vi "power_meas.vi"() -> ()   [LabVIEW 2019]
uses:
  <vilib>/Utility/error.llb/DialogType.ctl
  <vilib>/DAQmx/write.llb/DAQmx Write (Digital Bool 1Line 1Point).vi
  <vilib>/DAQmx/write.llb/DAQmx Write (Counter Frequency 1Chan 1Samp).vi
  <vilib>/DAQmx/miscellaneous.llb/DAQmx Fill In Error Info.vi
  <vilib>/DAQmx/create/channels.llb/DAQmx Create Channel (CO-Pulse Generation-Frequency).vi
  <vilib>/DAQmx/configure/timing.llb/DAQmx Timing (Implicit).vi
  <vilib>/addons/control/pid/pid.llb/PID (DBL).vi
  <vilib>/Utility/file.llb/Write Delimited Spreadsheet (string).vi
  <instrlib>/Agilent 34970/Agilent 34970.lvlib
  <resource>/objmgr/daqmx.rc
  <vilib>/addons/control/pid/NI_PID_pid.lvlib
  <instrlib>/Yokogawa WT200 Series/Yokogawa WT200 Series.lvlib
panel:
  in  "Idenfier_Ens. Term.":string="medsETMA"
  out "TP 15":dbl
  out "TP 13":dbl
  out "TP 12":dbl
  out "TP 11":dbl
  out "TP 10":dbl
  out "TP 8":dbl
  out "TP 7":dbl
  out "TP 6":dbl
  out "TP 5":dbl
  out "TP 3":dbl
  out "TP 2":dbl
  out "TP 1":dbl
  in  "Idenfier_Freio":string="medsFreio"
  in  "Identifier_Watt":string="medsWatt"
  out "PL(E)":dbl
  out "PC(E)":dbl
  out "PC(T)":dbl
  out "PL(T)":dbl
  out "t":dbl
  out "Tensão de saída":dbl format="%.4f"
  out "Corrente de saída":dbl format="%.4f"
  out "watt num cluster":T1
  in  "Liga Fonte":bool
  out "Resposta":string
  out "Tradução":string
  in  "Parar motor":bool
  in  "Envia mensagem":bool
  in  "Enviar velocidade":bool
  in  "Seta carga":bool
  in  "Limite de tensão":dbl=17.0 min=0.0 max=17.0 step=0.5 format="%.4f"
  in  "Limite de corrente":dbl=0.075 min=0.0 max=0.4 step=0.01 format="%.4f"
  in  "Mensagem":T2(ring)=enum."Read power"
  in  "Velocidade (RPM)":u16=1000 min=1000 max=10000 step=100
  in  "Parâmetros serial":T3={"Serial VCC"="COM7", "timeout"=2, "baud rate"=600, "flow control"=0, "data bits"=8, "parity"=enum."None", "stop bits"=10, "termination char"=FALSE} {"stop bits" items=["1.0"=10, "1.5"=15, "2.0"=20]; "flow control" items=["None", "XON/XOFF", "RTS/CTS", "XON/XOFF & RTS/CTS", "DTR/DSR", "XON/XOFF & DTR/DSR"]}
  in  "Medição contínua? WT230":bool=TRUE
  in  "Realiza medição WT230":bool=TRUE
  out "Chart potencia numeric":T4(graph)
  out "Chart corrente numeric":cluster{"I(A)":dbl, "I(B)":dbl, "I(E)":dbl}(graph)
  out "Chart tensão numeric":cluster{"V(A)":dbl, "V(B)":dbl, "V(E)":dbl}(graph)
  in  "Tempo de integração (s)":u32=5 min=1 max=60 step=1
  in  "SP:":dbl(slide)=25.0 min=0.0 max=0.0 scale=25.0..50.0
  out "MV":dbl(graph)
  in  "Ts":dbl=1.0
  out "PV":dbl
  out "Process variable and Setpoint":cluster{"initial PV":dbl, "SP:":dbl}(graph)
  in  "PID gains":T5={"proportional gain (Kc)"=39.6, "integral time (Ti, min)"=14.617, "derivative time (Td, min)"=0.0} {"derivative time (Td, min)" format="%.3f"; "integral time (Ti, min)" format="%.3f"; "proportional gain (Kc)" format="%.6f"}
  in  "Frequency":dbl=1.0 format="%.6f"
  out "Duty Cycle":sgl=0.1 min=0.1 max=99.9 format="%#_6f"
  in  "Forno_on":bool=TRUE
  out "Iteration":i32
  out "Chart PV, SP":cluster{dbl, dbl}(graph)
  in  "STOP":bool
  out "Temperature CH4 [degC]":dbl
  out "Temperature CH9 [degC]":dbl
  out "Time":dbl=300.0 format="%<%H:%M:%S>t"
  in  "Idenfier_Forno":string="medsForno"
  # "Temperaturas dos Termopares"
  # "Controle de Temperatura do Forno"
  # "Freio"
  # "Wattímetro WT230 Yokogawa"
  # "Geral"
  # "Respostas do Sistema em Malha Fechada"
  # "Controles"
  # "Controles"
  # "Medidas"
  # "Respostas temporais"
  # "Medidas"
  # "Controles"
  # "Inversor de Frequência"
  # "Comandos"
  # "Medidas"
  # "Parâmetros Serial"
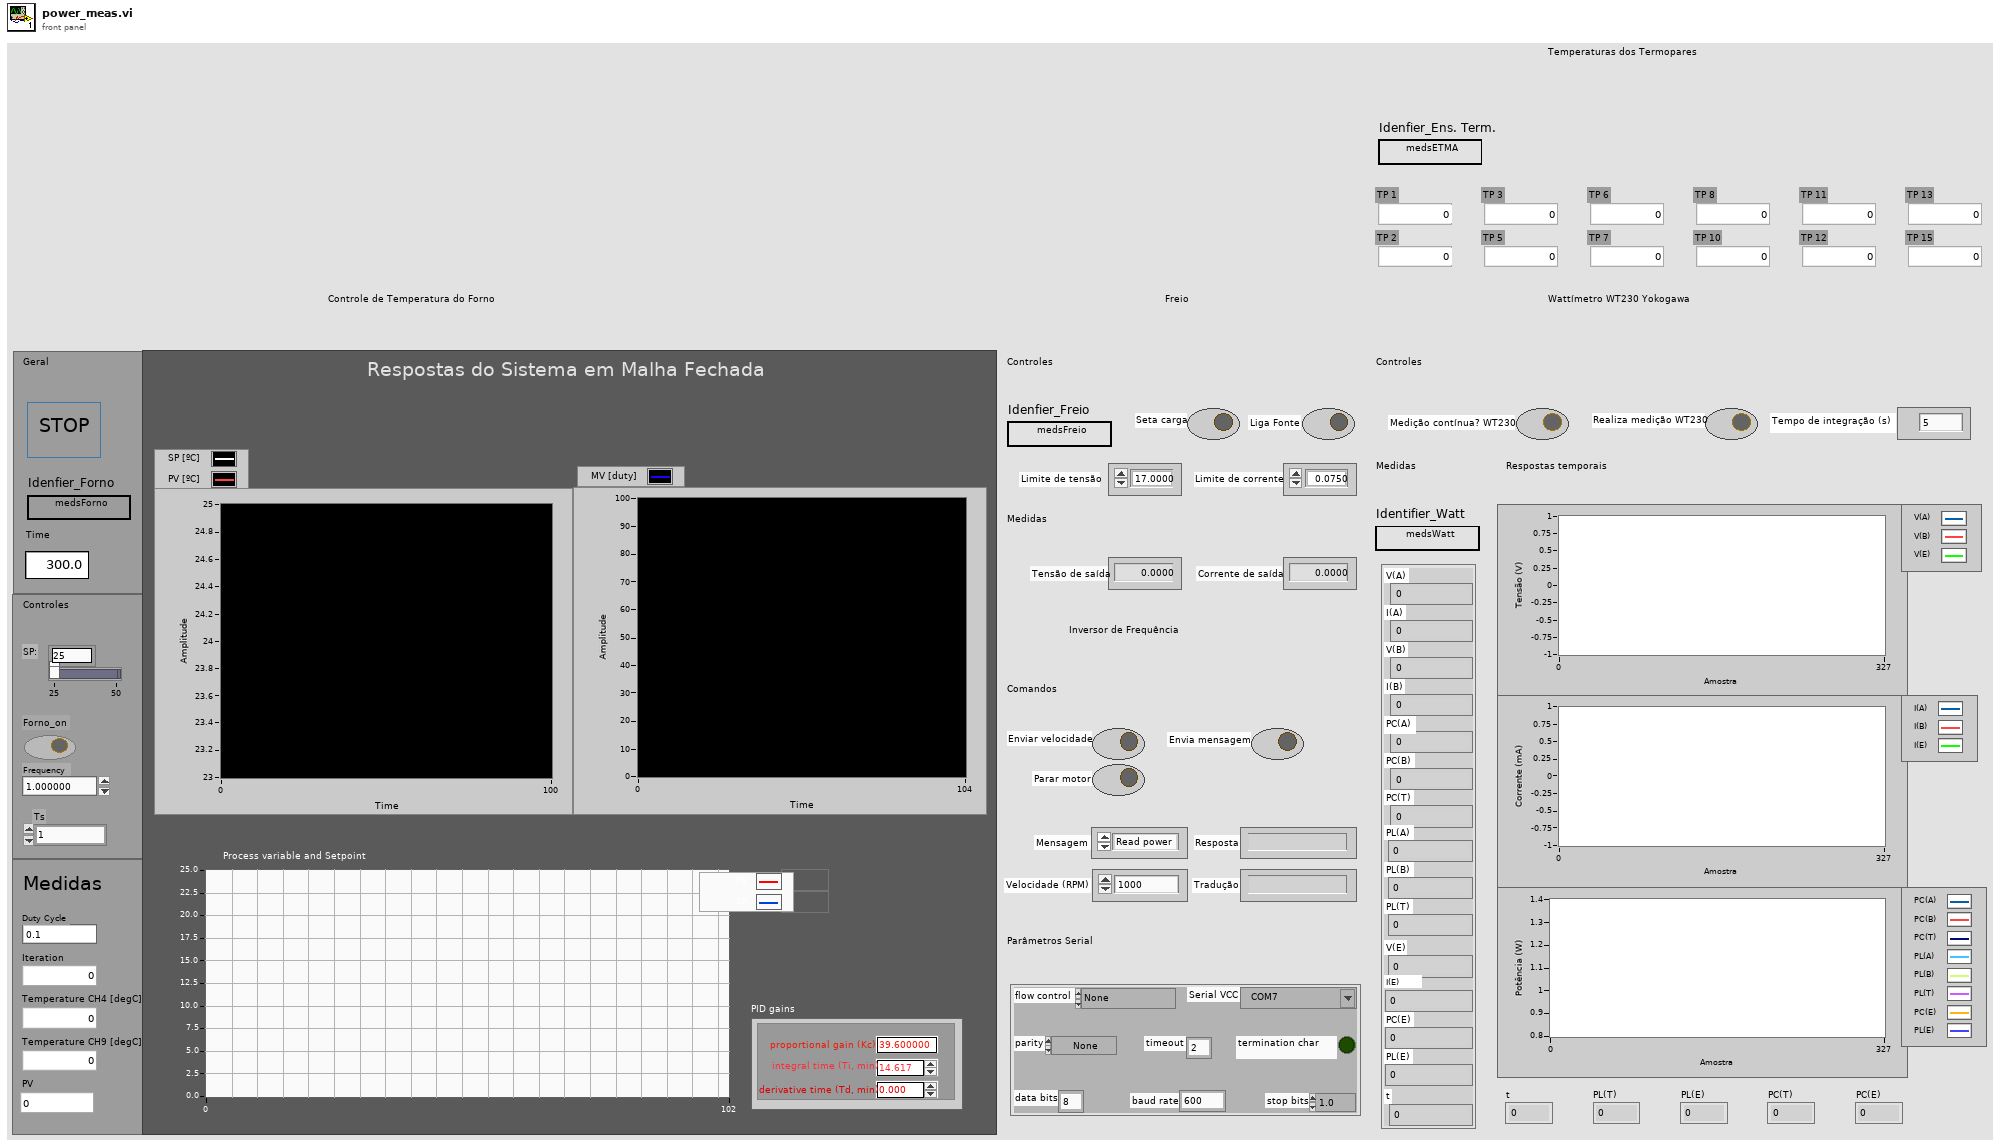
[diagram p1: front panel]
types:
  T1 = cluster{"V(A)":dbl, "I(A)":dbl, "V(B)":dbl, "I(B)":dbl, "PC(A)":dbl, "PC(B)":dbl, "PC(T)":dbl, "PL(T)":dbl, "PL(B)":dbl, "PL(A)":dbl, "V(E)":dbl, "PL(E)":dbl, "PC(E)":dbl, "I(E)":dbl, "t":dbl}
  T2 = enum16{"Read set speed", "Read operation status", "Read power", "Read starting trials", "Read bus voltage", "Read temperature", "Read power limitation", "Read PWM mode", "Read PWM frequency", "Read real speed"}
  T3 = cluster{"Serial VCC":refnum<visa-resource-name>, "timeout":u32, "baud rate":u32, "flow control":u16, "data bits":u16, "parity":enum16{"None", "Odd", "Even", "Mark", "Space"}, "stop bits":u16, "termination char":bool}
  T4 = cluster{"PC(A)":dbl, "PC(B)":dbl, "PC(T)":dbl, "PL(A)":dbl, "PL(B)":dbl, "PL(T)":dbl, "PC(E)":dbl, "PL(E)":dbl}
  T5 = cluster{"proportional gain (Kc)":dbl, "integral time (Ti, min)":dbl, "derivative time (Td, min)":dbl}
  T6 = enum16{"Start Comm.", "End Comm.", "Wait", "Send Static Message", "Set Speed"}
  T7 = enum16{"Thermocouple", "Thermistor", "RTD", "4-Wire RTD", "Default (Last)"}
  T8 = enum8{"Enabled", "Disabled", "Disabled and Grayed Out"}
  T9 = typedef "DialogType.ctl" = u16
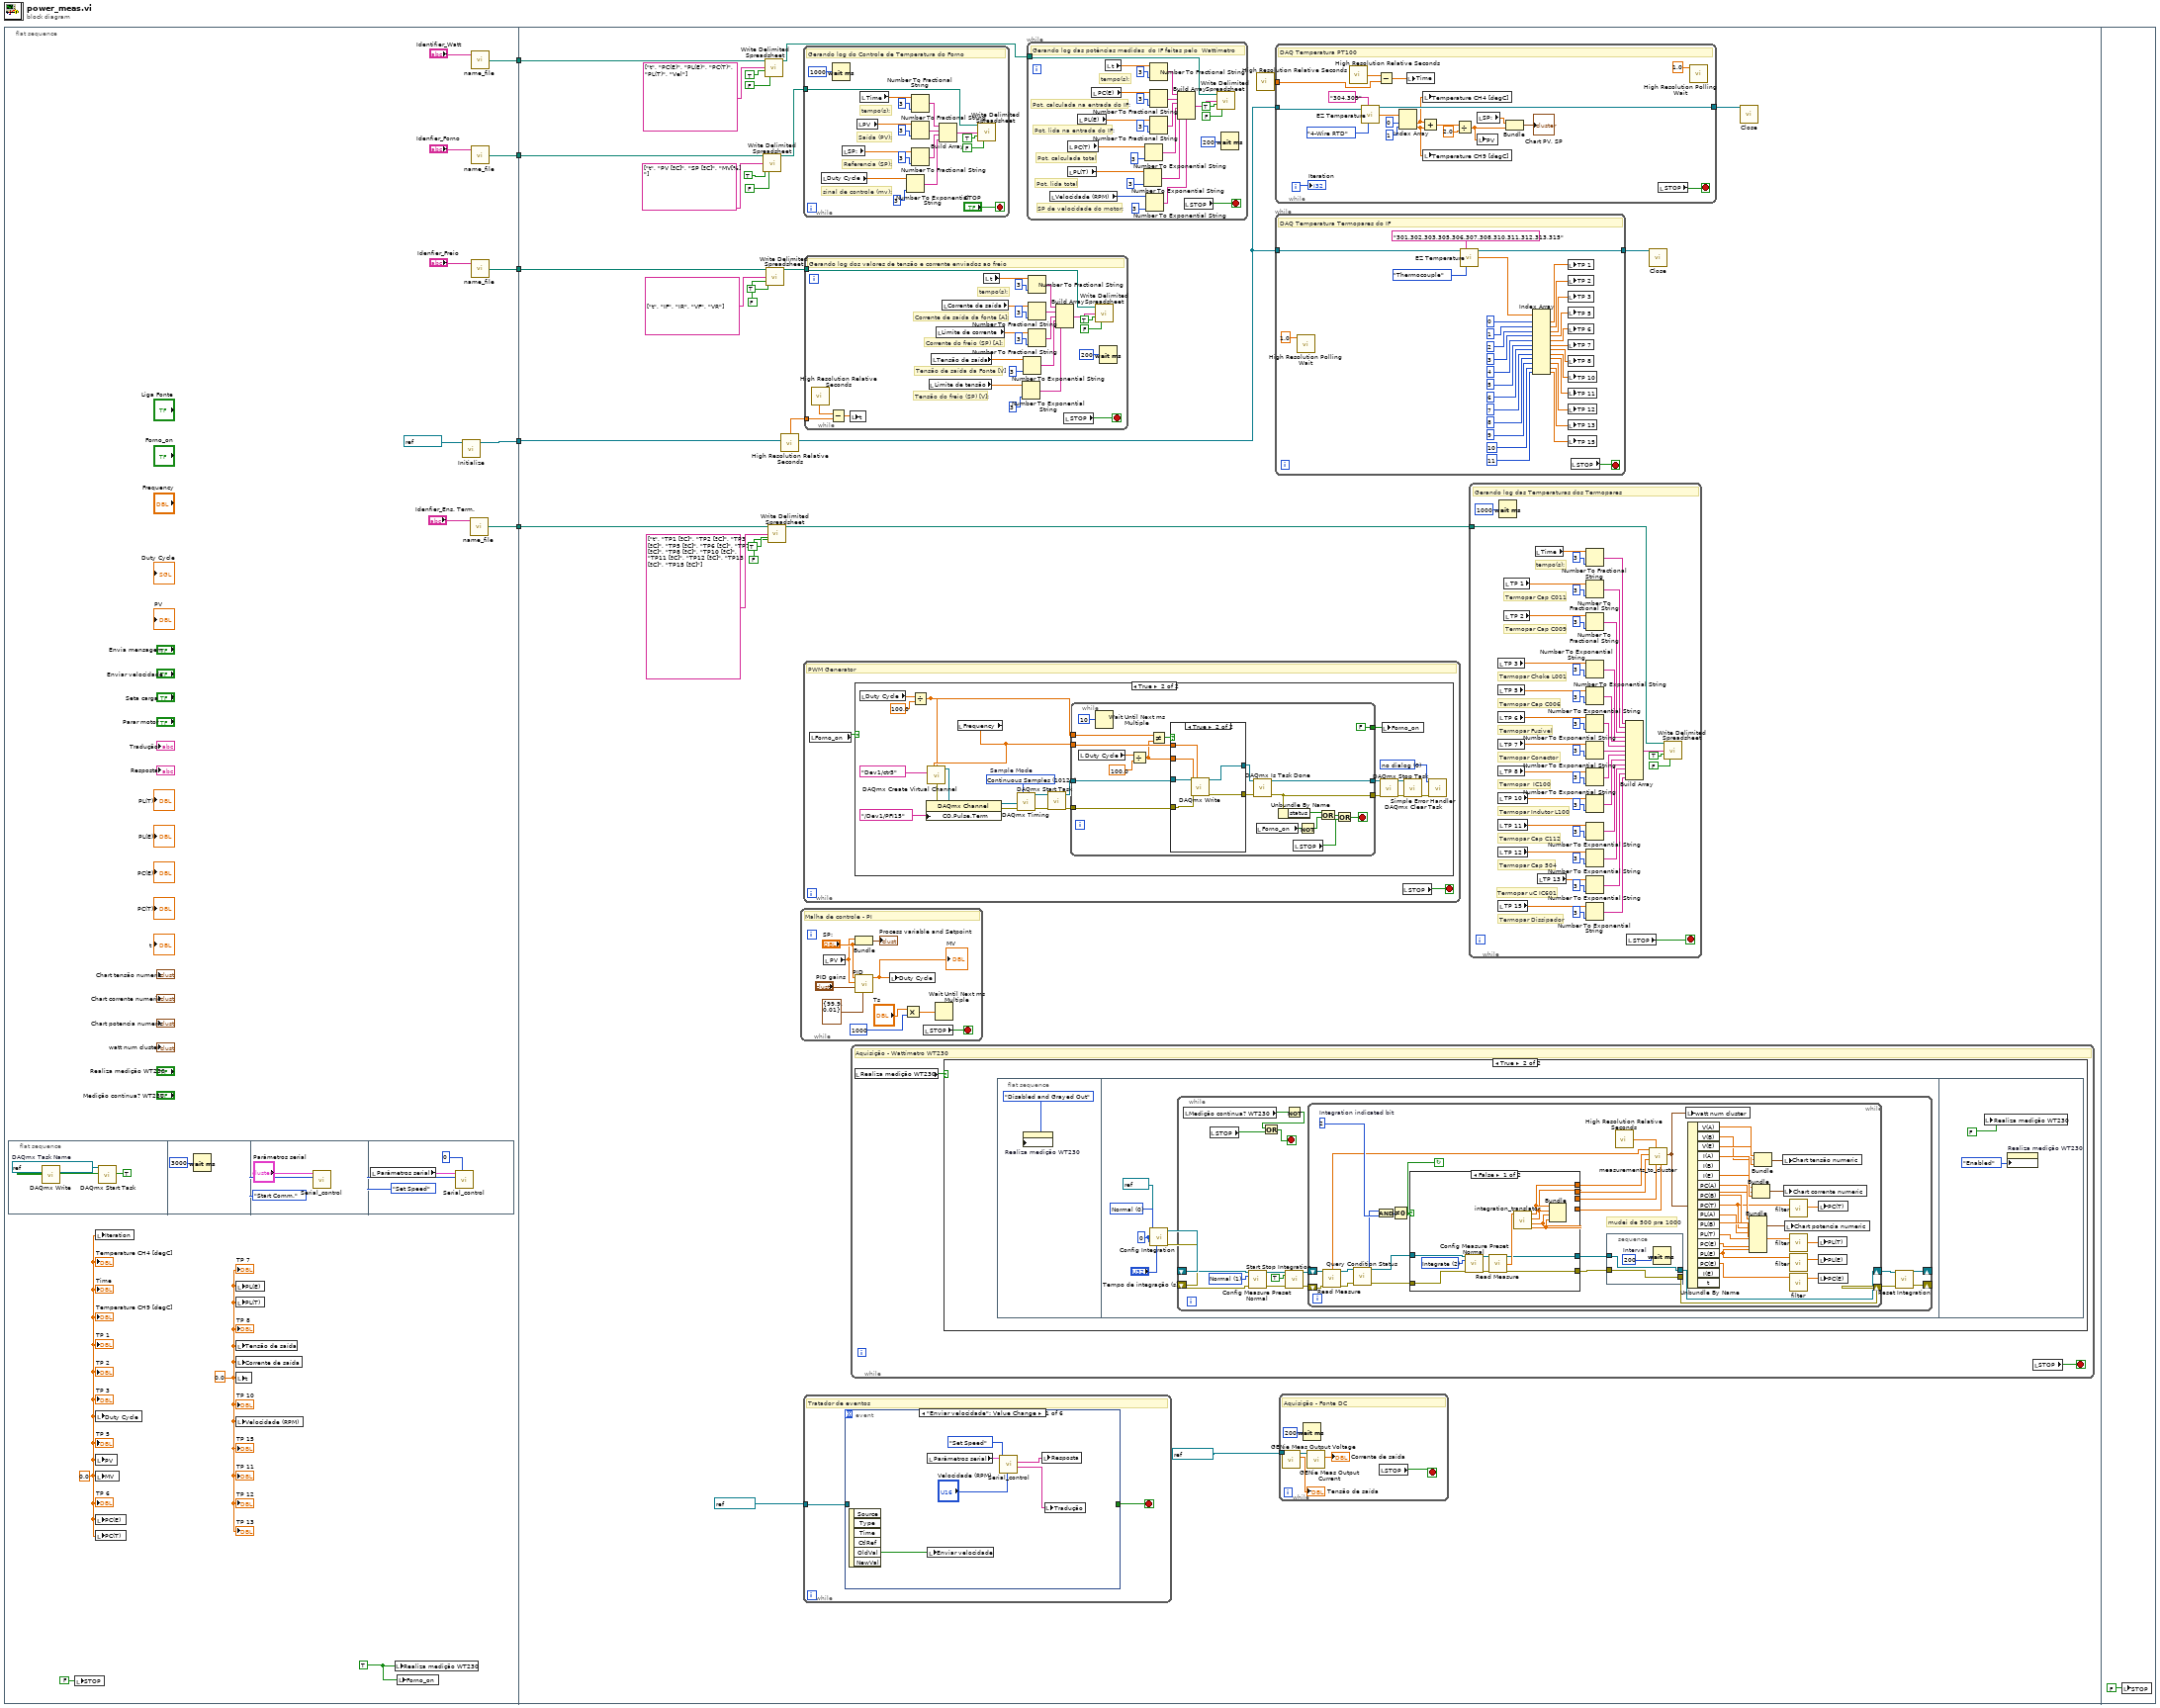
[diagram p0: block diagram]
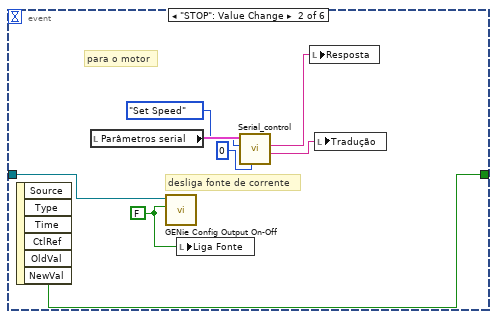
[diagram p2: hidden frame]
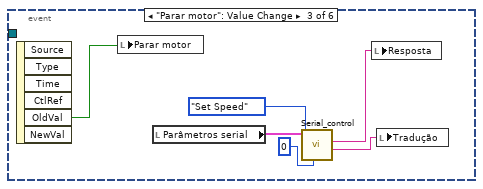
[diagram p3: hidden frame]
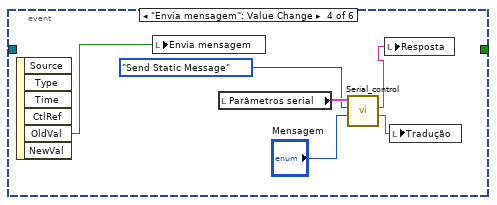
[diagram p4: hidden frame]
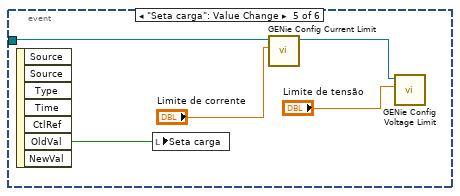
[diagram p5: hidden frame]
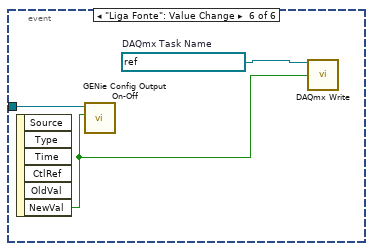
[diagram p6: hidden frame]
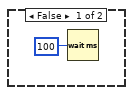
[diagram p7: hidden frame]
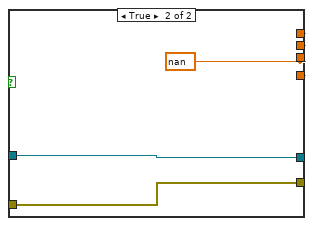
[diagram p8: hidden frame]
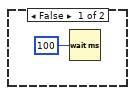
[diagram p9: hidden frame]
diagram:
  n1 = flat-sequence {
    tunnel: [w18] -> w5
    tunnel: [w17] -> w4
    tunnel: [w13] -> w3
    tunnel: [w11] -> w2
    tunnel: [w6] -> w1
    tunnel: w5 -> [w30]
    tunnel: w4 -> [w49]
    tunnel: w3 -> [w46]
    tunnel: w2 -> [w41]
    tunnel: w1 -> [w32]
    frame #0 {
      w8 = 0.0 ("Temperature 1")
      w10 = TRUE ("Realiza medição WT230")
      w9 = 0.0 ("Temperature 1")
      n2 = flat-sequence {
        frame #0 {
          w20 = refnum<k21> "alimentacao_inversor"  # DAQmx Task Name
          n3 = call <vilib>:"DAQmx Start Task.vi"("task/channels in"=w20) -> ("task out"=w22:refnum<k21>)  [unwired: 13 in, 1 out]
          n4 = call-poly <vilib>:"DAQmx Write.vi"("task/channels in"=w22, "data"=TRUE) -> ()  [unwired: 11 in, 3 out]
        }
        frame #1 {
          n5 = Wait (ms)(milliseconds to wait=u32 3000) -> ()  [unwired: 1 out]
        }
        frame #2 {
          n6 = call "Serial_control.vi"("Função"=T6."Start Comm.", "comm cluster"="Parâmetros serial") -> ()  [unwired: 3 in, 4 out]
        }
        frame #3 {
          n7 = local read "Parâmetros serial"() -> (w27:T3)
          n8 = call "Serial_control.vi"("Enviar número"=u16 0, "Função"=T6."Set Speed", "comm cluster"=w27) -> ()  [unwired: 2 in, 4 out]
        }
      }
      n9 = local write "STOP"(FALSE ("STOP")) -> ()
      n10 = local write "Iteration"(w9) -> ()
      n11 = local write "Duty Cycle"(w9) -> ()
      n12 = local write "PV"(w9) -> ()
      n13 = local write "MV"(w9) -> ()
      n14 = local write "PC(E)"(w9) -> ()
      n15 = local write "PC(T)"(w9) -> ()
      n16 = local write "PL(E)"(w8) -> ()
      n17 = local write "PL(T)"(w8) -> ()
      n18 = local write "Tensão de saída"(w8) -> ()
      n19 = local write "Corrente de saída"(w8) -> ()
      n20 = local write "t"(w8) -> ()
      n21 = local write "Velocidade (RPM)"(w8) -> ()
      n22 = local write "Realiza medição WT230"(w10) -> ()
      n23 = local write "Forno_on"(w10) -> ()
      n24 = call <instrlib>:"Initialize.vi"("VISA Resource Name"=refnum<visa-resource-name> "Agilent" ("VISA AGILENT")) -> ("VISA Resource Name Out"=w18:refnum<visa-resource-name>)  [unwired: 13 in, 1 out]
      n25 = call "name_file.vi"("Identifier"="Idenfier_Ens. Term.") -> ("appended path"=w6:path)  [unwired: 2 in]
      n26 = call "name_file.vi"("Identifier"="Identifier_Watt") -> ("appended path"=w13:path)  [unwired: 2 in]
      n27 = call "name_file.vi"("Identifier"="Idenfier_Forno") -> ("appended path"=w17:path)  [unwired: 2 in]
      n28 = call "name_file.vi"("Identifier"="Idenfier_Freio") -> ("appended path"=w11:path)  [unwired: 2 in]
      "Temperature CH4 [degC]" <- w9
      "Temperature CH9 [degC]" <- w9
      "Time" <- w9
      "TP 1" <- w9
      "TP 2" <- w9
      "TP 3" <- w9
      "TP 5" <- w9
      "TP 6" <- w9
      "TP 7" <- w8
      "TP 8" <- w8
      "TP 10" <- w8
      "TP 11" <- w8
      "TP 12" <- w8
      "TP 13" <- w8
      "TP 15" <- w8
    }
    frame #1 {
      n29 = call-poly <vilib>:"Write Delimited Spreadsheet.vi"("file path (dialog if empty)"=w49, "1D data"=string[] ["t", "PV [ºC]", "SP [ºC]", "MV[%] "] ("appended array"), "append to file? (new file:F)"=TRUE, "transpose? (no:F)"=FALSE) -> ("new file path (Not A Path if cancelled)"=w50:path)  [unwired: 10 in, 1 out]
      n30 = call-poly <vilib>:"Write Delimited Spreadsheet.vi"("file path (dialog if empty)"=w46, "1D data"=string[] ["t", "PC(E)", "PL(E)", "PC(T)", "PL(T)", "Vel"] ("appended array"), "append to file? (new file:F)"=TRUE, "transpose? (no:F)"=FALSE) -> ("new file path (Not A Path if cancelled)"=w42:path)  [unwired: 10 in, 1 out]
      n31 = call-poly <vilib>:"Write Delimited Spreadsheet.vi"("file path (dialog if empty)"=w41, "1D data"=string[] ["t", "IF", "IR", "VF", "VR"] ("appended array"), "append to file? (new file:F)"=TRUE, "transpose? (no:F)"=FALSE) -> ("new file path (Not A Path if cancelled)"=w37:path)  [unwired: 10 in, 1 out]
      n32 = call-poly <vilib>:"Write Delimited Spreadsheet.vi"("file path (dialog if empty)"=w32, "1D data"=string[] ["t", "TP1 [ºC]", "TP2 [ºC]", "TP3 [ºC]", "TP5 [ºC]", "TP6 [ºC]", "TP7 [ºC]", "TP8 [ºC]", "TP10 [ºC]", "TP11 [ºC]", "TP12 [ºC]", "TP13 [ºC]", "TP15 [ºC]"] ("appended array"), "append to file? (new file:F)"=TRUE, "transpose? (no:F)"=FALSE) -> ("new file path (Not A Path if cancelled)"=w31:path)  [unwired: 10 in, 1 out]
      n33 = call <vilib>:"High Resolution Relative Seconds.vi"() -> ("relative seconds"=w36:dbl)
      n34 = while {
        stop <- w313 stop-if-true
        # "Malha de controle - PI"
        n35 = local read "PV"() -> (w317:dbl)
        n36 = Bundle("PV"=w317, "SP:"="SP:") -> (→"Process variable and Setpoint":cluster{"PV":dbl, "SP:":dbl})  [unwired: 1 in]
        n37 = call-poly <vilib>:"PID.vi"("output range"=cluster{"output high":dbl, "output low":dbl} {"output high"=99.9, "output low"=0.01}, "PID gains"="PID gains", "process variable"=w317, "setpoint"="SP:") -> ("output"=w312:dbl)  [unwired: 6 in, 1 out]
        "MV" <- w312
        n38 = local write "Duty Cycle"(w312) -> ()
        n39 = Multiply(x="Ts", y=u32 1000 ("unsigned 32bit integer")) -> (x*y=w311:dbl)
        n40 = local read "STOP"() -> (w313:bool)
        n41 = Wait Until Next ms Multiple(millisecond multiple=w311) -> ()  [unwired: 1 out]
      }
      n42 = while {
        tunnel: w50 -> [w389]
        stop <- "STOP" stop-if-true
        # "tempo(s):"
        # "Saída (PV):"
        # "Referencia (SP):"
        # "sinal de controle (mv):"
        # "Gerando log do Controle de Temperatura do Forno"
        n43 = local read "Duty Cycle"() -> (w385:sgl)
        n44 = Wait (ms)(milliseconds to wait=u32 1000) -> ()  [unwired: 1 out]
        n45 = local read "SP:"() -> (w378:dbl)
        n46 = local read "PV"() -> (w384:dbl)
        n47 = local read "Time"() -> (w382:dbl)
        n48 = Number To Exponential String(number=w385, precision (6)=i16 3) -> (E-format string=w387:string)  [unwired: 2 in]
        n49 = Number To Fractional String(number=w382, precision (6)=i16 3) -> (F-format string=w381:string)  [unwired: 2 in]
        n50 = Number To Fractional String(number=w384, precision (6)=i16 3) -> (F-format string=w380:string)  [unwired: 2 in]
        n51 = Number To Fractional String(number=w378, precision (6)=i16 3) -> (F-format string=w376:string)  [unwired: 2 in]
        n52 = Build Array(w381, w380, w376, w387) -> (w377:string[])
        n53 = call-poly <vilib>:"Write Delimited Spreadsheet.vi"("file path (dialog if empty)"=w389, "1D data"=w377, "append to file? (new file:F)"=TRUE, "transpose? (no:F)"=FALSE) -> ()  [unwired: 10 in, 2 out]
      }
      n54 = while {
        stop <- w321 stop-if-true
        # "PWM Generator"
        n55 = local read "Forno_on"() -> (w322:bool)
        n56 = case shown="True" w322 {
          frame False {
            n57 = Wait (ms)(milliseconds to wait=u32 100) -> ()  [unwired: 1 out]
          }
          frame True {
            w330 = T9 0 items=["no dialog", "OK message", "continue or stop message", "OK message + warnings", "continue/stop + warnings"] ("type of dialog (OK msg:1)")
            w341 = 10123 items=["Finite Samples"=10178, "Continuous Samples"=10123, "Hardware Timed Single Point"=12522]  # Sample Mode
            n58 = local read "Duty Cycle"() -> (w325:sgl)
            n59 = Divide(x=w325, y=100.0) -> (x/y=w324:dbl)
            n60 = local read "Frequency"() -> (w327:dbl)
            n61 = call-poly <vilib>:"DAQmx Create Virtual Channel.vi"("frequency"=w327, "duty cycle"=w324, "counter"=tag "Dev1/ctr3" ("Counter")) -> ("task out"=w344:refnum<k21>, "error out"=w343:errorcluster)  [unwired: 11 in]
            n62 = property class="DAQmx Channel"(reference=w344, error in=w343, "CO.Pulse.Term"=tag "/Dev1/PFI15" ("Output Terminal")) -> (reference out=w340:refnum<k21>, error out=w339:errorcluster)
            n63 = call-poly <vilib>:"DAQmx Timing.vi"("task/channels in"=w340, "sample mode"=w341, "error in"=w339) -> ("task out"=w338:refnum<k21>, "error out"=w337:errorcluster)  [unwired: 11 in]
            n64 = call <vilib>:"DAQmx Start Task.vi"("task/channels in"=w338, "error in"=w337) -> ("task out"=w336:refnum<k21>, "error out"=w335:errorcluster)  [unwired: 12 in]
            n65 = while {
              tunnel: w336 -> [w355]
              tunnel: w335 -> [w353]
              tunnel: [w364] -> w332
              tunnel: [w365] -> w333
              tunnel: [FALSE ("Liga aquecedor")] -> w329
              tunnel: w324 -> [w351]
              tunnel: w327 -> [w349]
              stop <- w358 stop-if-true
              n66 = local read "Duty Cycle"() -> (w348:sgl)
              n67 = Wait Until Next ms Multiple(millisecond multiple=u32 10) -> ()  [unwired: 1 out]
              n68 = Divide(x=w348, y=100.0) -> (x/y=w346:dbl)
              n69 = Not Equal?(x=w351, y=w346) -> (x != y?=w350:bool)
              n70 = case shown="True" w350 {
                tunnel: [w367 w370] -> w354
                tunnel: w355 -> [w367 w371]
                tunnel: [w366 w372] -> w352
                tunnel: w353 -> [w366 w373]
                tunnel: w346 -> [_ w369]
                tunnel: w349 -> [_ w368]
                frame False {
                }
                frame True {
                  n71 = call-poly <vilib>:"DAQmx Write.vi"("task/channels in"=w371, "frequency"=w368, "duty cycle"=w369, "error in"=w373) -> ("task out"=w370:refnum<k21>, "error out"=w372:errorcluster)  [unwired: 9 in, 1 out]
                }
              }
              n72 = call <vilib>:"DAQmx Is Task Done.vi"("task/channels in"=w354, "error in"=w352) -> ("task out"=w365:refnum<k21>, "error out"=w364:errorcluster)  [unwired: 11 in, 1 out]
              n73 = local read "Forno_on"() -> (w361:bool)
              n74 = Unbundle By Name(w364) -> ("status"=w363:bool)
              n75 = local read "STOP"() -> (w356:bool)
              n76 = Not(x=w361) -> (.not. x?=w359:bool)
              n77 = Or(x=w363, y=w359) -> (x .or. y?=w357:bool)
              n78 = Or(x=w357, y=w356) -> (x .or. y?=w358:bool)
            }
            n79 = call <vilib>:"DAQmx Stop Task.vi"("task/channels in"=w333, "error in"=w332) -> ("task out"=w328:refnum<k21>, "error out"=w334:errorcluster)  [unwired: 12 in]
            n80 = local write "Forno_on"(w329) -> ()
            n81 = call <vilib>:"DAQmx Clear Task.vi"("task in"=w328, "error in"=w334) -> ("error out"=w331:errorcluster)  [unwired: 13 in]
            n82 = call <vilib>:"Simple Error Handler.vi"("error code (no error:0)"=w330, "error in (no error)"=w331) -> ()  [unwired: 3 in, 5 out]
          }
        }
        n83 = local read "STOP"() -> (w321:bool)
      }
      n84 = while {
        tunnel: refnum<visa-resource-name> "Lambda" ("VISA name") -> [w186]
        stop <- w187 stop-if-true
        # "Tratador de eventos"
        n85 = event shown="[0] \"Enviar velocidade\": Value Change" {
          selector: _ -> [_ _ _ _ _ _]
          dyn-events: _ -> [_ _ _ _ _ _]
          timeout: _ -> [_ _ _ _ _ _]
          tunnel: w186 -> [_ w195 _ _ w215 w221]
          tunnel: [_ w196 _ _ _ _] -> w187
          event "Enviar velocidade": Value Change {
            n86 = event-data() -> ("OldVal"=w193:bool)  [unwired: 1 in, 5 out]
            n87 = local read "Parâmetros serial"() -> (w192:T3)
            n88 = local write "Enviar velocidade"(w193) -> ()
            n89 = call "Serial_control.vi"("Enviar número"="Velocidade (RPM)", "Função"=T6."Set Speed", "comm cluster"=w192) -> ("translated message"=w189:string, "read buffer"=w190:string)  [unwired: 2 in, 2 out]
            n90 = local write "Resposta"(w190) -> ()
            n91 = local write "Tradução"(w189) -> ()
          }
          event "STOP": Value Change {
            w194 = FALSE ("Output ON")
            # "desliga fonte de corrente"
            # "para o motor"
            n92 = event-data() -> ("NewVal"=w196:bool)  [unwired: 1 in, 5 out]
            n93 = local read "Parâmetros serial"() -> (w201:T3)
            n94 = call <instrlib>:"GENie Config Output On-Off.vi"("Output ON"=w194, "VISA"=w195) -> ()  [unwired: 8 in, 2 out]
            n95 = local write "Liga Fonte"(w194) -> ()
            n96 = call "Serial_control.vi"("Enviar número"=u16 0, "Função"=T6."Set Speed", "comm cluster"=w201) -> ("translated message"=w199:string, "read buffer"=w200:string)  [unwired: 2 in, 2 out]
            n97 = local write "Resposta"(w200) -> ()
            n98 = local write "Tradução"(w199) -> ()
          }
          event "Parar motor": Value Change {
            n99 = event-data() -> ("OldVal"=w204:bool)  [unwired: 1 in, 5 out]
            n100 = local write "Parar motor"(w204) -> ()
            n101 = local read "Parâmetros serial"() -> (w207:T3)
            n102 = call "Serial_control.vi"("Enviar número"=u16 0, "Função"=T6."Set Speed", "comm cluster"=w207) -> ("translated message"=w202:string, "read buffer"=w203:string)  [unwired: 2 in, 2 out]
            n103 = local write "Resposta"(w203) -> ()
            n104 = local write "Tradução"(w202) -> ()
          }
          event "Envia mensagem": Value Change {
            n105 = event-data() -> ("OldVal"=w213:bool)  [unwired: 1 in, 5 out]
            n106 = local write "Envia mensagem"(w213) -> ()
            n107 = local read "Parâmetros serial"() -> (w212:T3)
            n108 = call "Serial_control.vi"("Message"="Mensagem", "Função"=T6."Send Static Message", "comm cluster"=w212) -> ("translated message"=w210:string, "read buffer"=w209:string)  [unwired: 2 in, 2 out]
            n109 = local write "Resposta"(w209) -> ()
            n110 = local write "Tradução"(w210) -> ()
          }
          event "Seta carga": Value Change {
            n111 = event-data() -> ("OldVal"=w216:bool)  [unwired: 1 in, 6 out]
            n112 = local write "Seta carga"(w216) -> ()
            n113 = call <instrlib>:"GENie Config Current Limit.vi"("Current Limit"="Limite de corrente", "VISA"=w215) -> ("VISA out"=w214:refnum<visa-resource-name>)  [unwired: 8 in, 1 out]
            n114 = call <instrlib>:"GENie Config Voltage Limit.vi"("Volt Limit"="Limite de tensão", "VISA"=w214) -> ()  [unwired: 8 in, 2 out]
          }
          event "Liga Fonte": Value Change {
            w220 = refnum<k21> "resfriamento_freio"  # DAQmx Task Name
            n115 = event-data() -> ("NewVal"=w219:bool)  [unwired: 1 in, 5 out]
            n116 = call <instrlib>:"GENie Config Output On-Off.vi"("Output ON"=w219, "VISA"=w221) -> ()  [unwired: 8 in, 2 out]
            n117 = call-poly <vilib>:"DAQmx Write.vi"("task/channels in"=w220, "data"=w219) -> ()  [unwired: 11 in, 3 out]
          }
        }
      }
      n118 = while {
        tunnel: w37 -> [w153]
        tunnel: w36 -> [w133]
        stop <- w139 stop-if-true
        # "Tensão do freio (SP) [V]:"
        # "tempo(s):"
        # "Corrente de saída da fonte [A]:"
        # "Corrente do freio (SP) [A]:"
        # "Tensão de saída da Fonte [V]"
        # "Gerando log dos valores de tensão e corrente enviados ao freio"
        n119 = call <vilib>:"High Resolution Relative Seconds.vi"() -> ("relative seconds"=w134:dbl)
        n120 = Subtract(x=w134, y=w133) -> (x-y=w132:dbl)
        n121 = local write "t"(w132) -> ()
        n122 = local read "Limite de tensão"() -> (w137:dbl)
        n123 = local read "Tensão de saída"() -> (w149:dbl)
        n124 = local read "Limite de corrente"() -> (w142:dbl)
        n125 = local read "Corrente de saída"() -> (w148:dbl)
        n126 = local read "t"() -> (w146:dbl)
        n127 = Number To Exponential String(number=w137, precision (6)=i16 3) -> (E-format string=w135:string)  [unwired: 2 in]
        n128 = Number To Exponential String(number=w149, precision (6)=i16 3) -> (E-format string=w151:string)  [unwired: 2 in]
        n129 = Number To Fractional String(number=w146, precision (6)=i16 3) -> (F-format string=w145:string)  [unwired: 2 in]
        n130 = Number To Fractional String(number=w148, precision (6)=i16 3) -> (F-format string=w144:string)  [unwired: 2 in]
        n131 = Number To Fractional String(number=w142, precision (6)=i16 3) -> (F-format string=w140:string)  [unwired: 2 in]
        n132 = Build Array(w145, w144, w140, w151, w135) -> (w141:string[])
        n133 = local read "STOP"() -> (w139:bool)
        n134 = call-poly <vilib>:"Write Delimited Spreadsheet.vi"("file path (dialog if empty)"=w153, "1D data"=w141, "append to file? (new file:F)"=TRUE, "transpose? (no:F)"=FALSE) -> ()  [unwired: 10 in, 2 out]
        n135 = Wait (ms)(milliseconds to wait=u32 200) -> ()  [unwired: 1 out]
      }
      n136 = while {
        stop <- w222 stop-if-true
        # "Aquisição - Wattímetro WT230"
        n137 = local read "Realiza medição WT230"() -> (w223:bool)
        n138 = case shown="True" w223 {
          frame False {
            n139 = Wait (ms)(milliseconds to wait=u32 100) -> ()  [unwired: 1 out]
          }
          frame True {
            n140 = flat-sequence {
              frame #0 {
                n141 = property on="Realiza medição WT230" class="Bool (strict)"("DisabledEnum"=T8."Disabled and Grayed Out" ("Disabled")) -> ()  [unwired: 2 in, 2 out]
              }
              frame #1 {
                w228 = u16 0 items=["Normal", "Continuous"] ("Integ Mode (0: Normal)")
                w229 = u32 0 ("Hour (0)")
                n142 = call <instrlib>:"Config Integration.vi"("VISA resource name"=refnum<visa-resource-name> "WT", "Integ Mode (0: Normal)"=w228, "Hour (0)"=w229, "Minute (0)"=w229, "Second (0)"="Tempo de integração (s)") -> ("VISA resource name out"=w231:refnum<visa-resource-name>, "error out"=w230:errorcluster)  [unwired: 9 in]
                n143 = while {
                  shift-right: [w235] -> _
                  shift-left: w231 -> [w233]
                  shift-right: [w234] -> _
                  shift-left: w230 -> [w232]
                  stop <- w236 stop-if-true
                  w242 = u16 1 items=["Clear", "Normal", "Integrate"] ("Preset Pattern (0: Clear)")
                  n144 = local read "Medição contínua? WT230"() -> (w238:bool)
                  n145 = local read "STOP"() -> (w239:bool)
                  n146 = call <instrlib>:"Config Measure Preset Normal.vi"("VISA resource name"=w233, "Preset Pattern (0: Clear)"=w242, "error in (no error)"=w232) -> ("VISA resource name out"=w244:refnum<visa-resource-name>, "error out"=w243:errorcluster)  [unwired: 11 in]
                  n147 = Not(x=w238) -> (.not. x?=w237:bool)
                  n148 = Or(x=w237, y=w239) -> (x .or. y?=w236:bool)
                  n149 = call <instrlib>:"Start Stop Integration.vi"("VISA resource name"=w244, "Start/Stop (F: Stop)"=TRUE, "error in (no error)"=w243) -> ("VISA resource name out"=w247:refnum<visa-resource-name>, "error out"=w246:errorcluster)  [unwired: 11 in]
                  n150 = while {
                    shift-left: w247 -> [w287]
                    shift-right: [w275] -> w241
                    shift-left: w246 -> [w284]
                    shift-right: [w273] -> w240
                    stop <- w283 continue-if-true
                    w290 = u16 2  # Integration indicated bit
                    # "mudei de 500 pra 1000"
                    n151 = call <instrlib>:"Read Measure.vi"("VISA resource name"=w287, "error in (no error)"=w284) -> ("VISA resource name out"=w286:refnum<visa-resource-name>, "Measure Value"=w277:sgl[], "error out"=w285:errorcluster)  [unwired: 10 in, 1 out]
                    n152 = call <instrlib>:"Query Condition Status.vi"("VISA resource name"=w286, "error in (no error)"=w285) -> ("VISA resource name out"=w272:refnum<visa-resource-name>, "Condition"=w288:u16, "error out"=w271:errorcluster)  [unwired: 11 in]
                    n153 = And(x=w288, y=w290) -> (x .and. y?=w289:u16)
                    n154 = Not Equal To 0?(x=w289) -> (x != 0?=w283:bool)
                    n155 = case shown="False" w283 {
                      tunnel: [w301 w308] -> w282
                      tunnel: [w300 w308] -> w281
                      tunnel: [w299 w308] -> w280
                      tunnel: [w298 w308] -> w279
                      tunnel: [w297 w307] -> w276
                      tunnel: [w296 w306] -> w274
                      tunnel: w272 -> [w295 w307]
                      tunnel: w271 -> [w294 w306]
                      frame False {
                        w302 = u16 2 items=["Clear", "Normal", "Integrate"] ("Preset Pattern (0: Clear)")
                        n156 = call <instrlib>:"Config Measure Preset Normal.vi"("VISA resource name"=w295, "Preset Pattern (0: Clear)"=w302, "error in (no error)"=w294) -> ("VISA resource name out"=w305:refnum<visa-resource-name>, "error out"=w304:errorcluster)  [unwired: 11 in]
                        n157 = call <instrlib>:"Read Measure.vi"("VISA resource name"=w305, "error in (no error)"=w304) -> ("VISA resource name out"=w297:refnum<visa-resource-name>, "Measure Value"=w303:sgl[], "error out"=w296:errorcluster)  [unwired: 10 in, 1 out]
                        n158 = call "integration_translator.vi"("Valores integração"=w303) -> ("PI(E)"=w298:sgl, "PI(T)"=w299:sgl, "PI(B)"=w300:sgl, "PI(A)"=w301:sgl)  [unwired: 7 in]
                        n159 = Bundle("PI(A)"=w301, "PI(B)"=w300, "PI(T)"=w299, "PI(E)"=w298) -> ()  [unwired: 1 in, 1 out]
                      }
                      frame True {
                        w308 = nan
                      }
                    }
                    n160 = stacked-sequence {
                      tunnel: w276 -> [w292]
                      tunnel: [w292] -> w275
                      tunnel: w274 -> [w291]
                      tunnel: [w291] -> w273
                      frame #0 {
                        w293 = u32 200  # Interval
                        n161 = Wait (ms)(milliseconds to wait=w293) -> ()  [unwired: 1 out]
                      }
                    }
                    n162 = call <vilib>:"High Resolution Relative Seconds.vi"() -> ("relative seconds"=w278:dbl)
                    n163 = call "measurements_to_cluster.vi"("PI(E)"=w279, "PI(T)"=w280, "relative seconds"=w278, "PI(B)"=w281, "PI(A)"=w282, "Measure Value"=w277) -> ("watt cluster"=w259:T1)  [unwired: 4 in, 1 out]
                    n164 = local write "watt num cluster"(w259) -> ()
                    n165 = Unbundle By Name(w259) -> ("V(A)"=w270:dbl, "V(B)"=w260:dbl, "V(E)"=w261:dbl, "I(A)"=w262:dbl, "I(B)"=w263:dbl, "I(E)"=w264:dbl, "PC(A)"=w265:dbl, "PC(B)"=w266:dbl, "PC(T)"=w255:dbl, "PL(A)"=w267:dbl, "PL(B)"=w268:dbl, "PL(T)"=w252:dbl, "PC(E)"=w269:dbl, "PL(E)"=w251:dbl, "PC(E)"=w249:dbl)  [unwired: 2 out]
                    n166 = Bundle("PC(A)"=w265, "PC(B)"=w266, "PC(T)"=w255, "PL(A)"=w267, "PL(B)"=w268, "PL(T)"=w252, "PC(E)"=w269, "PL(E)"=w251) -> (w257:T4)  [unwired: 1 in]
                    n167 = Bundle("I(A)"=w262, "I(B)"=w263, "I(E)"=w264) -> (w256:cluster{"I(A)":dbl, "I(B)":dbl, "I(E)":dbl})  [unwired: 1 in]
                    n168 = Bundle("V(A)"=w270, "V(B)"=w260, "V(E)"=w261) -> (w258:cluster{"V(A)":dbl, "V(B)":dbl, "V(E)":dbl})  [unwired: 1 in]
                    n169 = local write "Chart tensão numeric"(w258) -> ()
                    n170 = local write "Chart corrente numeric"(w256) -> ()
                    n171 = local write "Chart potencia numeric"(w257) -> ()
                    n172 = call "filter.vi"("input"=w255) -> ("output"=w254:dbl)  [unwired: 10 in]
                    n173 = call "filter.vi"("input"=w252) -> ("output"=w253:dbl)  [unwired: 10 in]
                    n174 = call "filter.vi"("input"=w251) -> ("output"=w250:dbl)  [unwired: 10 in]
                    n175 = call "filter.vi"("input"=w249) -> ("output"=w248:dbl)  [unwired: 10 in]
                    n176 = local write "PC(T)"(w254) -> ()
                    n177 = local write "PL(T)"(w253) -> ()
                    n178 = local write "PL(E)"(w250) -> ()
                    n179 = local write "PC(E)"(w248) -> ()
                  }
                  n180 = call <instrlib>:"Reset Integration.vi"("VISA resource name"=w241, "error in (no error)"=w240) -> ("VISA resource name out"=w235:refnum<visa-resource-name>, "error out"=w234:errorcluster)  [unwired: 12 in]
                }
              }
              frame #2 {
                n181 = local write "Realiza medição WT230"(FALSE ("Realiza medição")) -> ()
                n182 = property on="Realiza medição WT230" class="Bool (strict)"("DisabledEnum"=T8."Enabled" ("Disabled")) -> ()  [unwired: 2 in, 2 out]
              }
            }
          }
        }
        n183 = local read "STOP"() -> (w222:bool)
      }
      n184 = while {
        tunnel: w42 -> [w177]
        stop <- w163 stop-if-true
        # "SP de velocidade do motor:"
        # "Pot. lida total"
        # "tempo(s):"
        # "Pot. calculada na entrada do IF:"
        # "Pot. lida na entrada do IF:"
        # "Pot. calculada total"
        # "Gerando log das potências medidas  do IF feitas pelo  Wattímetro"
        n185 = local read "Velocidade (RPM)"() -> (w159:u16)
        n186 = local read "PL(T)"() -> (w162:dbl)
        n187 = local read "PC(T)"() -> (w173:dbl)
        n188 = local read "PL(E)"() -> (w166:dbl)
        n189 = local read "PC(E)"() -> (w172:dbl)
        n190 = local read "t"() -> (w170:dbl)
        n191 = Number To Exponential String(number=w162, precision (6)=i16 3) -> (E-format string=w160:string)  [unwired: 2 in]
        n192 = Number To Exponential String(number=w173, precision (6)=i16 3) -> (E-format string=w175:string)  [unwired: 2 in]
        n193 = Number To Exponential String(number=w159, precision (6)=i16 3) -> (E-format string=w156:string)  [unwired: 2 in]
        n194 = Number To Fractional String(number=w170, precision (6)=i16 3) -> (F-format string=w169:string)  [unwired: 2 in]
        n195 = Number To Fractional String(number=w172, precision (6)=i16 3) -> (F-format string=w168:string)  [unwired: 2 in]
        n196 = Number To Fractional String(number=w166, precision (6)=i16 3) -> (F-format string=w164:string)  [unwired: 2 in]
        n197 = Build Array(w169, w168, w164, w175, w160, w156) -> (w165:string[])
        n198 = local read "STOP"() -> (w163:bool)
        n199 = call-poly <vilib>:"Write Delimited Spreadsheet.vi"("file path (dialog if empty)"=w177, "1D data"=w165, "append to file? (new file:F)"=TRUE, "transpose? (no:F)"=FALSE) -> ()  [unwired: 10 in, 2 out]
        n200 = Wait (ms)(milliseconds to wait=u32 200) -> ()  [unwired: 1 out]
      }
      n201 = call <vilib>:"High Resolution Relative Seconds.vi"() -> ("relative seconds"=w55:dbl)
      n202 = while {
        tunnel: w30 -> [w393]
        tunnel: w55 -> [w395]
        tunnel: [w409] -> w54
        i -> [w410]
        stop <- w392 stop-if-true
        # "DAQ Temperatura PT100"
        n203 = call <vilib>:"High Resolution Relative Seconds.vi"() -> ("relative seconds"=w394:dbl)
        n204 = call <instrlib>:"EZ Temperature.vi"("VISA Resource Name"=w393, "Scan List (empty)"="304,309", "Transducer Type (4:Def-Last)"=T7."4-Wire RTD") -> ("VISA Resource Name Out"=w409:refnum<visa-resource-name>, "Output Array"=w403:dbl[])  [unwired: 10 in, 1 out]
        n205 = Subtract(x=w394, y=w395) -> (x-y=w404:dbl)
        n206 = Index Array(array=w403, index #1=0 ("index"), index #2=1 ("index")) -> (element #1=w396:dbl, element #2=w397:dbl)
        n207 = local write "Time"(w404) -> ()
        n208 = Add(x=w396, y=w397) -> (x+y=w402:dbl)
        n209 = local write "Temperature CH4 [degC]"(w396) -> ()
        n210 = local write "Temperature CH9 [degC]"(w397) -> ()
        n211 = Divide(x=w402, y=2.0) -> (x/y=w399:dbl)
        n212 = local read "SP:"() -> (w400:dbl)
        n213 = local write "PV"(w399) -> ()
        n214 = Bundle("SP:"=w400, w399) -> (→"Chart PV, SP":cluster{"SP:":dbl, dbl})  [unwired: 1 in]
        n215 = local read "STOP"() -> (w392:bool)
        n216 = call <vilib>:"High Resolution Polling Wait.vi"("seconds to wait"=1.0) -> ()  [unwired: 10 in, 1 out]
        "Iteration" <- w410
      }
      n217 = while {
        tunnel: w30 -> [w58]
        tunnel: [w56] -> w29
        stop <- w60 stop-if-true
        # "DAQ Temperatura Termopares do IF"
        n218 = call <vilib>:"High Resolution Polling Wait.vi"("seconds to wait"=1.0) -> ()  [unwired: 10 in, 1 out]
        n219 = call <instrlib>:"EZ Temperature.vi"("VISA Resource Name"=w58, "Scan List (empty)"="301,302,303,305,306,307,308,310,311,312,313,315", "Transducer Type (4:Def-Last)"=T7."Thermocouple") -> ("VISA Resource Name Out"=w56:refnum<visa-resource-name>, "Output Array"=w63:dbl[])  [unwired: 10 in, 1 out]
        n220 = Index Array(array=w63, index #1=0 ("index"), index #2=1 ("index"), index #3=2 ("index"), index #4=3 ("index"), index #5=4 ("index"), index #6=5 ("index"), index #7=6 ("index"), index #8=7 ("index"), index #9=8 ("index"), index #10=9 ("index"), index #11=10 ("index"), index #12=11 ("index")) -> (element #1=w75:dbl, element #2=w76:dbl, element #3=w77:dbl, element #4=w78:dbl, element #5=w79:dbl, element #6=w80:dbl, element #7=w81:dbl, element #8=w82:dbl, element #9=w83:dbl, element #10=w84:dbl, element #11=w85:dbl, element #12=w86:dbl)
        n221 = local write "TP 1"(w75) -> ()
        n222 = local write "TP 2"(w76) -> ()
        n223 = local write "TP 3"(w77) -> ()
        n224 = local write "TP 5"(w78) -> ()
        n225 = local write "TP 6"(w79) -> ()
        n226 = local write "TP 7"(w80) -> ()
        n227 = local write "TP 8"(w81) -> ()
        n228 = local write "TP 10"(w82) -> ()
        n229 = local write "TP 11"(w83) -> ()
        n230 = local write "TP 12"(w84) -> ()
        n231 = local write "TP 13"(w85) -> ()
        n232 = local write "TP 15"(w86) -> ()
        n233 = local read "STOP"() -> (w60:bool)
      }
      n234 = while {
        tunnel: refnum<visa-resource-name> "Lambda" ("VISA name") -> [w181]
        stop <- w180 stop-if-true
        # "Aquisição - Fonte DC"
        n235 = call <instrlib>:"GENie Meas Output Voltage.vi"("VISA"=w181) -> ("Output Voltage"=→"Tensão de saída":dbl, "VISA out"=w184:refnum<visa-resource-name>)  [unwired: 8 in, 1 out]
        n236 = Wait (ms)(milliseconds to wait=u32 200) -> ()  [unwired: 1 out]
        n237 = call <instrlib>:"GENie Meas Output Current.vi"("VISA"=w184) -> ("Output Current"=→"Corrente de saída":dbl)  [unwired: 8 in, 2 out]
        n238 = local read "STOP"() -> (w180:bool)
      }
      n239 = while {
        tunnel: w31 -> [w129]
        stop <- w115 stop-if-true
        # "Termopar Dissipador"
        # "Termopar uC IC601"
        # "Termopar Cap 504"
        # "Termopar Cap C112"
        # "Termopar Indutor L100"
        # "Termopar  IC100"
        # "Termopar Conector"
        # "Termopar Fusivel"
        # "Termopar Cap C006"
        # "tempo(s):"
        # "Termopar Cap C011"
        # "Termopar Cap C009"
        # "Termopar Choke L001"
        # "Gerando log das Temperaturas dos Termopares"
        n240 = local read "TP 3"() -> (w125:dbl)
        n241 = local read "TP 5"() -> (w112:dbl)
        n242 = local read "TP 6"() -> (w111:dbl)
        n243 = local read "TP 7"() -> (w108:dbl)
        n244 = local read "TP 8"() -> (w107:dbl)
        n245 = local read "TP 10"() -> (w104:dbl)
        n246 = local read "TP 11"() -> (w103:dbl)
        n247 = local read "TP 12"() -> (w100:dbl)
        n248 = local read "TP 15"() -> (w97:dbl)
        n249 = Wait (ms)(milliseconds to wait=u32 1000) -> ()  [unwired: 1 out]
        n250 = local read "TP 1"() -> (w114:dbl)
        n251 = local read "TP 2"() -> (w119:dbl)
        n252 = local read "Time"() -> (w123:dbl)
        n253 = local read "TP 13"() -> (w99:dbl)
        n254 = Number To Fractional String(number=w123, precision (6)=i16 3) -> (F-format string=w122:string)  [unwired: 2 in]
        n255 = Number To Fractional String(number=w114, precision (6)=i16 3) -> (F-format string=w121:string)  [unwired: 2 in]
        n256 = Number To Fractional String(number=w119, precision (6)=i16 3) -> (F-format string=w117:string)  [unwired: 2 in]
        n257 = Number To Exponential String(number=w125, precision (6)=i16 3) -> (E-format string=w127:string)  [unwired: 2 in]
        n258 = Number To Exponential String(number=w112, precision (6)=i16 3) -> (E-format string=w96:string)  [unwired: 2 in]
        n259 = Number To Exponential String(number=w111, precision (6)=i16 3) -> (E-format string=w95:string)  [unwired: 2 in]
        n260 = Number To Exponential String(number=w108, precision (6)=i16 3) -> (E-format string=w94:string)  [unwired: 2 in]
        n261 = Number To Exponential String(number=w107, precision (6)=i16 3) -> (E-format string=w93:string)  [unwired: 2 in]
        n262 = Number To Exponential String(number=w104, precision (6)=i16 3) -> (E-format string=w92:string)  [unwired: 2 in]
        n263 = Number To Exponential String(number=w103, precision (6)=i16 3) -> (E-format string=w91:string)  [unwired: 2 in]
        n264 = Number To Exponential String(number=w100, precision (6)=i16 3) -> (E-format string=w90:string)  [unwired: 2 in]
        n265 = Number To Exponential String(number=w99, precision (6)=i16 3) -> (E-format string=w89:string)  [unwired: 2 in]
        n266 = Number To Exponential String(number=w97, precision (6)=i16 3) -> (E-format string=w88:string)  [unwired: 2 in]
        n267 = Build Array(w122, w121, w117, w127, w96, w95, w94, w93, w92, w91, w90, w89, w88) -> (w118:string[])
        n268 = local read "STOP"() -> (w115:bool)
        n269 = call-poly <vilib>:"Write Delimited Spreadsheet.vi"("file path (dialog if empty)"=w129, "1D data"=w118, "append to file? (new file:F)"=TRUE, "transpose? (no:F)"=FALSE) -> ()  [unwired: 10 in, 2 out]
      }
      n270 = call <instrlib>:"Close.vi"("VISA Resource Name"=w29) -> ()  [unwired: 14 in, 1 out]
      n271 = call <instrlib>:"Close.vi"("VISA Resource Name"=w54) -> ()  [unwired: 14 in, 1 out]
    }
    frame #2 {
      n272 = local write "STOP"(FALSE ("STOP")) -> ()
    }
  }
